vi "util_BuildPWMParams.vi"(0 "Burst":bool, 5 "Continous":bool, 7 "Frequency (Hz)":dbl=10000.0, 9 "Amplitude (V)":dbl, 11 "Duty Cycle (0-1)":dbl=0.5) -> (4 "PWM Params":T1={"Pulse Length (Ticks)"=4294967295, "Pulse Period (Ticks)"=4294967295, "Ao (Int)"=0, "Seq 1 (High)"=TRUE, "Seq 2 (Low)"=TRUE})   [LabVIEW 2012]
panel:
  in  "Scaffold":T1
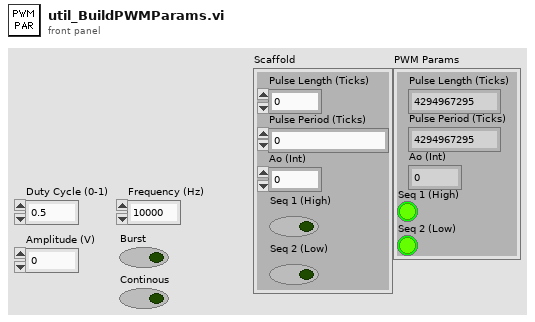
[diagram p1: front panel]
types:
  T1 = cluster{"Pulse Length (Ticks)":u32, "Pulse Period (Ticks)":u32, "Ao (Int)":i32, "Seq 1 (High)":bool, "Seq 2 (Low)":bool}
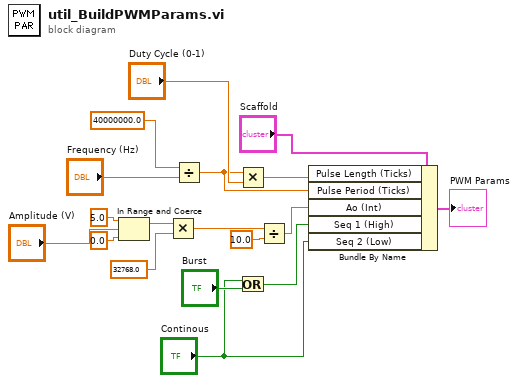
[diagram p0: block diagram]
diagram:
  n1 = In Range and Coerce(upper limit=5.0, x="Amplitude (V)", lower limit=0.0) -> (coerced(x)=w9:dbl)  [unwired: 1 out]
  n2 = Multiply(x=w9, y=32768.0) -> (x*y=w14:dbl)
  n3 = Divide(x=40000000.0, y="Frequency (Hz)") -> (x/y=w6:dbl)
  n4 = Multiply(x=w6, y="Duty Cycle (0-1)") -> (x*y=w5:dbl)
  n5 = Or(x="Continous", y="Burst") -> (x .or. y?=w3:bool)
  n6 = Divide(x=w14, y=10.0) -> (x/y=w4:dbl)
  n7 = Bundle By Name(cluster="Scaffold", "Pulse Length (Ticks)"=w5, "Pulse Period (Ticks)"=w6, "Ao (Int)"=w4, "Seq 1 (High)"=w3, "Seq 2 (Low)"="Continous") -> (→"PWM Params":T1)
